vi "libssh2_channel_open_session.vi"(8 "error in (no error)":errorcluster, 11 "Session":T1) -> (0 "error out":errorcluster, 3 "Channel":T2)   [LabVIEW 2013, in "libssh2.lvlib"]
uses:
  libssh2.lvlib
  Channel Refnum.ctl
  Session Refnum.ctl
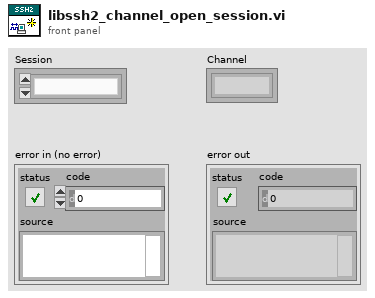
[diagram p1: front panel]
types:
  T1 = typedef "libssh2.lvlib/Session Refnum.ctl" = refnum<k1>
  T2 = typedef "libssh2.lvlib/Channel Refnum.ctl" = refnum<k1>
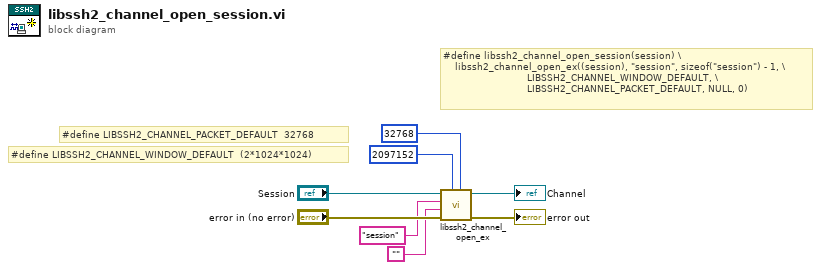
[diagram p0: block diagram]
diagram:
  # "#define LIBSSH2_CHANNEL_PACKET_DEFAULT  32768"
  # "#define LIBSSH2_CHANNEL_WINDOW_DEFAULT  (2*1024*1024)"
  # "#define libssh2_channel_open_session(session) \\\n    libssh2_channel_open_ex((session), \"session\", sizeof(\"session\") - 1, \\\n                            LIBSSH2_CHANNEL_WINDOW_DEFAULT, \\\n                            LIBSSH2_CHANNEL_PACKET_DEFAULT, NULL, 0)"
  n1 = call "libssh2_channel_open_ex.vi"("packet_size"=u32 32768, "window_size"=u32 2097152, "error in (no error)"="error in (no error)", "message"="", "channel_type"="session", "Session"="Session") -> ("error out"=→"error out":errorcluster, "Channel"=→"Channel":T2)  [unwired: 4 in]
